vi "Write Sense_Point.vi"(8 "error in":errorcluster, 10 "Sense Point":T1, 11 "89XX in":refnum<class "89XX.lvclass">) -> (0 "error out":errorcluster, 3 "89XX out":refnum<class "89XX.lvclass">)   [LabVIEW 2019, in "89XX.lvlib" / "89XX.lvclass"]
uses:
  Library/89XX.lvclass
  C:/Users/Public/Documents/Development/builds/Instruments/PowerSupply.lvlibp/Library/PowerSupply.lvclass
  C:/Users/Public/Documents/Development/builds/Engine/Monitored Actor.lvlibp/Monitored Actor/Monitored Actor/Monitored Actor.lvclass
  builds/Instruments/PowerSupply.lvlibp/Custom Controls/Sense Point.ctl
  builds/Engine/Monitored Actor.lvlibp/Monitored Actor/Monitored Actor/Read Actor Label.vi
  <vilib>/ErrorRing/Error Ring.xnode
  builds/Instruments/PowerSupply.lvlibp/Library/PowerSupply.lvclass
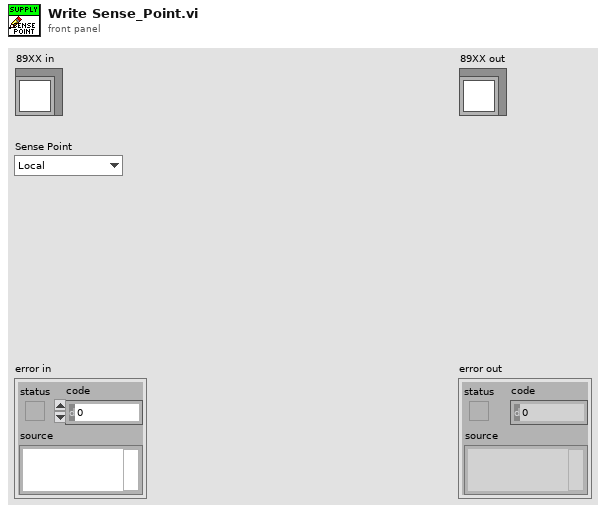
[diagram p1: front panel]
types:
  T1 = typedef "PowerSupply.lvlibp/PowerSupply.lvclass/Sense Point.ctl" = enum16{"Local", "Remote"}
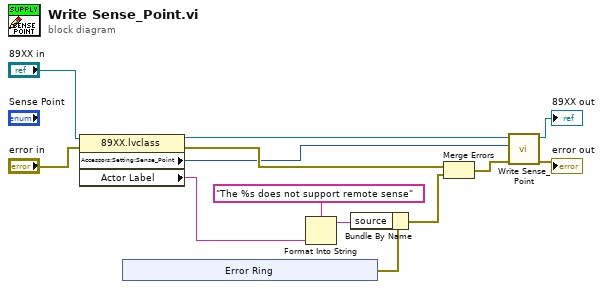
[diagram p0: block diagram]
diagram:
  n1 = property class="89XX.lvclass"(reference="89XX in", error in="error in") -> (reference out=w5:refnum<class "89XX.lvclass">, error out=w13:errorcluster, "Accessors:Setting:Sense_Point"=w1:T1, "Actor Label"=w9:string)
  n2 = xnode "Error Ring"() -> ("error out"=w12:errorcluster)
  n3 = Format Into String(format string="The %s does not support remote sense", w9) -> (resulting string=w11:string)  [unwired: 2 in, 1 out]
  n4 = Bundle By Name(cluster=w12, "source"=w11) -> (w10:errorcluster)
  n5 = Merge Errors(w13, w10) -> (w2:errorcluster)
  n6 = call-parent "Write Sense_Point.vi"("error in"=w2, "Sense Point"=w1, "PowerSupply in"=w5) -> ("error out"=→"error out":errorcluster, "PowerSupply out"=→"89XX out":refnum<class "89XX.lvclass">)  [unwired: 7 in]
